vi "Write Anthropic_key.vi"(8 "error in (no error)":errorcluster, 10 "Anthropic_key":string, 11 "llm_anthropic_chatmodels in":refnum<class "llm_anthropic_chatmodels.lvclass">) -> (0 "error out":errorcluster, 3 "llm_anthropic_chatmodels out":refnum<class "llm_anthropic_chatmodels.lvclass">)   [LabVIEW 2020, in "llm_anthropic_chatmodels.lvclass"]
uses:
  llm_anthropic_chatmodels.lvclass
  llm_anthropic_chatmodels.lvclass/llm_anthropic_chatmodels.ctl
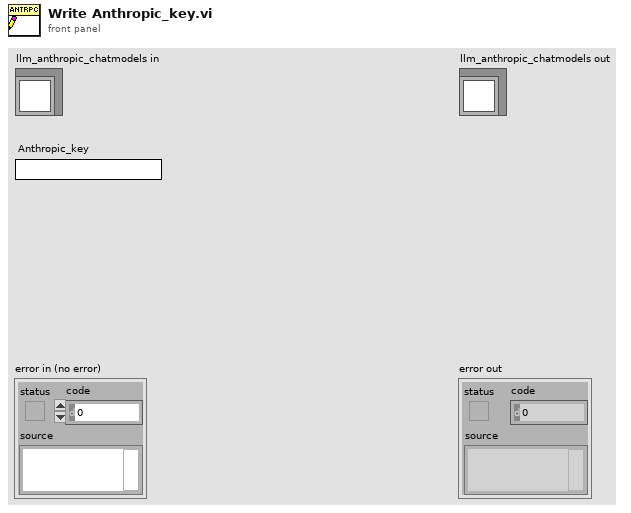
[diagram p1: front panel]
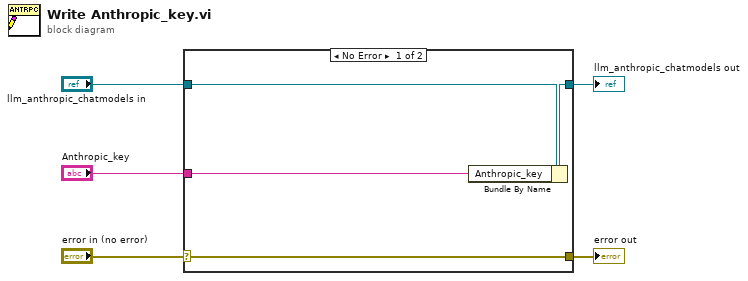
[diagram p0: block diagram]
diagram:
  n1 = case shown="No Error" "error in (no error)" {
    selector: "error in (no error)" -> [w9 w10]
    tunnel: [w9 w10] -> w4
    tunnel: [w7 w11] -> w2
    tunnel: "llm_anthropic_chatmodels in" -> [w8 w11]
    tunnel: "Anthropic_key" -> [w6 _]
    frame No Error {
      n2 = Bundle By Name(cluster=w8, "Anthropic_key"=w6) -> (w7:refnum<class "llm_anthropic_chatmodels.lvclass">)
    }
    frame Error {
    }
  }
  "error out" <- w4
  "llm_anthropic_chatmodels out" <- w2
